vi "rdb_json_load.vi"(7 "type":variant, 8 "error in (no error)":errorcluster, 10 "strict validation? (F)":bool, 11 "json":string) -> (0 "error out":errorcluster, 2 "elements":T1[](array[typedef]), 3 "value":variant)   [LabVIEW 2017]
uses:
  rdb_json_element.ctl
  rdb_json_type.ctl
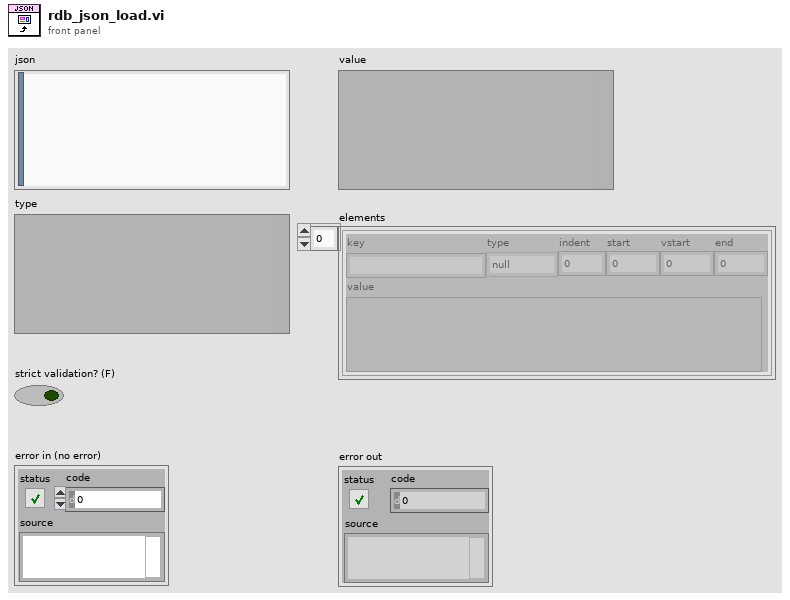
[diagram p1: front panel]
types:
  T1 = typedef "rdb_json_element.ctl" = cluster{"key":string, "type":T2, "indent":i32, "start":i32, "vstart":i32, "end":i32, "value":variant}
  T2 = typedef "rdb_json_type.ctl" = enum8{"null", "bool", "int", "uint", "float", "string", "array", "object", "invalid"}
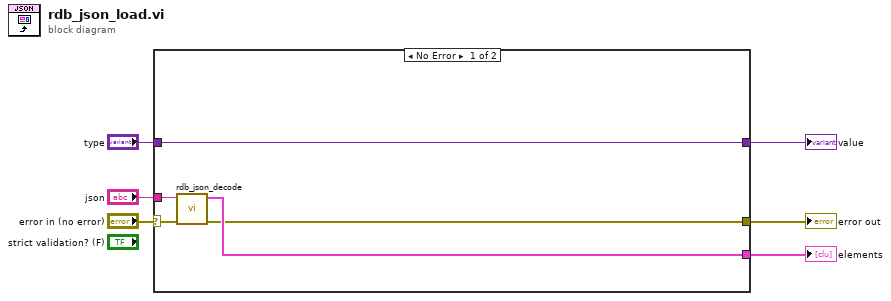
[diagram p0: block diagram]
diagram:
  n1 = case shown="No Error" "error in (no error)" {
    selector: "error in (no error)" -> [w11 w13]
    tunnel: "json" -> [w10 _]
    tunnel: [w7 w13] -> w4
    tunnel: [w9 w12] -> w3
    tunnel: "type" -> [w9 w12]
    tunnel: [w8 _] -> w1
    frame No Error {
      n2 = call "rdb_json_decode.vi"("error in (no error)"=w11, "json"=w10) -> ("error out"=w7:errorcluster, "elements"=w8:T1[])  [unwired: 8 in]
    }
    frame Error {
    }
  }
  "error out" <- w4
  "value" <- w3
  "elements" <- w1
